vi "ReadConfig.vi"(8 "error in (no error)":errorcluster, 11 "GRMActor in":refnum<class "MicroscopeController.lvclass">) -> (0 "error out":errorcluster, 3 "GRMActor out":refnum<class "MicroscopeController.lvclass">)   [LabVIEW 2020, in "MicroscopeController.lvlib" / "MicroscopeController.lvclass"]
uses:
  MicroscopeController.lvclass
  MicroscopeController.lvclass/MicroscopeController.ctl
  Model/Hardware Abstraction Layer/Component/GenericActor/GenericActor/GenericController.lvclass
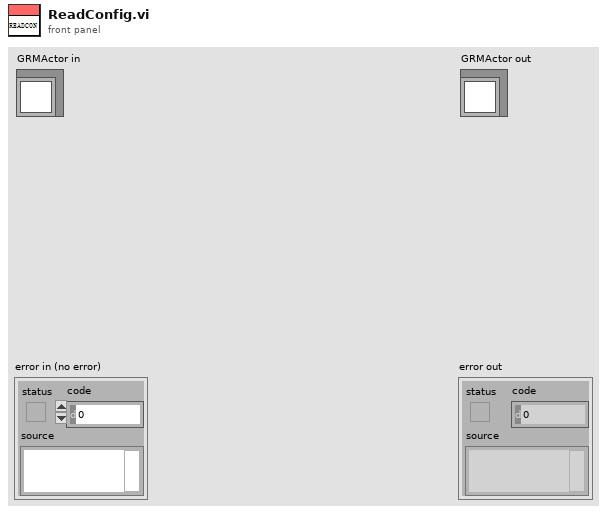
[diagram p1: front panel]
types:
  T1 = typedef "NI_LVConfig.lvlib/Config Data RefNum.ctl" = refnum<k1>
  T2 = cluster{"Values[0]":i32, "Values[1]":i32, "Values[2]":i32, "Values[3]":i32}
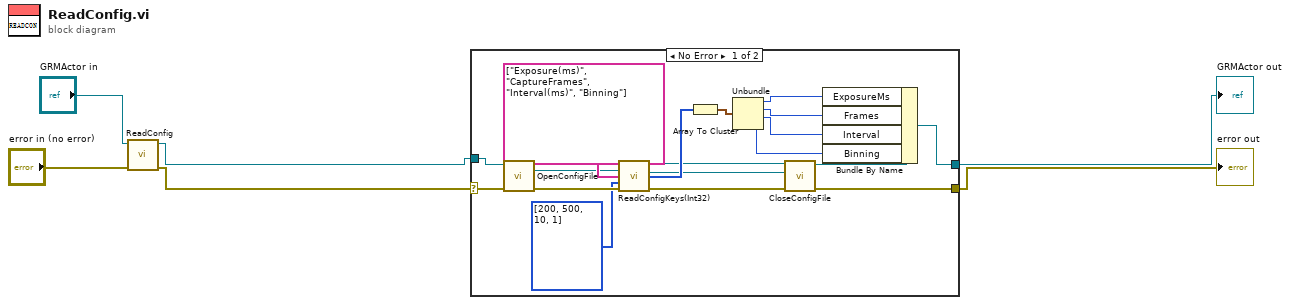
[diagram p0: block diagram]
diagram:
  n1 = call-parent "ReadConfig.vi"("error in (no error)"="error in (no error)", "GRMActor in"="GRMActor in") -> ("error out"=w3:errorcluster, "GRMActor out"=w4:refnum<class "MicroscopeController.lvclass">)  [unwired: 8 in]
  n2 = case shown="No Error" w3 {
    selector: w3 -> [w25 w26]
    tunnel: [w11 w26] -> w1
    tunnel: [w19 w27] -> w2
    tunnel: w4 -> [w24 w27]
    frame No Error {
      n3 = call-dynamic "OpenConfigFile.vi"("error in (no error)"=w25, "GRMActor in"=w24) -> ("error out"=w23:errorcluster, "refnum"=w13:T1, "GRMActor out"=w21:refnum<class "MicroscopeController.lvclass">)  [unwired: 7 in]
      n4 = call-dynamic "ReadConfigKeys(Int32).vi"("GRMActor in"=w21, "Config Refnum"=w13, "Keys"=string[] ["Exposure(ms)", "CaptureFrames", "Interval(ms)", "Binning"], "Default"=i32[] [200, 500, 10, 1], "error in (no error)"=w23) -> ("GRMActor out"=w10:refnum<class "MicroscopeController.lvclass">, "Config Refnum dup"=w8:T1, "Values"=w12:i32[], "error out"=w22:errorcluster)  [unwired: 7 in]
      n5 = Array To Cluster(array=w12) -> (cluster=w18:T2)
      n6 = Unbundle(w18) -> ("Values[0]"=w17:i32, "Values[1]"=w16:i32, "Values[2]"=w15:i32, "Values[3]"=w7:i32)
      n7 = call-dynamic "CloseConfigFile.vi"("error in (no error)"=w22, "refnum"=w8, "GRMActor in"=w10) -> ("error out"=w11:errorcluster, "GRMActor out"=w9:refnum<class "MicroscopeController.lvclass">)  [unwired: 7 in]
      n8 = Bundle By Name(cluster=w9, "ExposureMs"=w17, "Frames"=w16, "Interval"=w15, "Binning"=w7) -> (w19:refnum<class "MicroscopeController.lvclass">)
    }
    frame Error {
    }
  }
  "error out" <- w1
  "GRMActor out" <- w2
